vi "syncDAQ_branch.vi"() -> ()   [LabVIEW 2013]
uses:
  <vilib>/Utility/error.llb/DialogType.ctl
  <vilib>/DAQmx/read.llb/DAQmx Read (Analog 1D DBL 1Chan NSamp).vi
  <vilib>/DAQmx/read.llb/DAQmx Read (Analog 1D Wfm NChan NSamp).vi
  <vilib>/DAQmx/miscellaneous.llb/DAQmx Fill In Error Info.vi
  <vilib>/ErrorRing/Error Ring.xnode
panel:
  in  "Ratio":dbl=0.2 caption="复位时间比"
  in  "Vx_Max":dbl=3.0 caption="X向最大电压"
  in  "Vy_Max":dbl=3.0 caption="Y向最大电压"
  in  "N_x":i32=512 caption="采样行数"
  in  "N_y":i32=512 caption="每行采样数"
  in  "停止按钮":bool
  in  "每次采集行数":i32=16
  in  "physical channels read":tag="Dev1/ai0" caption="物理通道（读取）"
  in  "physical channels write":tag="Dev1/ao0:1" caption="物理通道（写入）"
  out "number of samples\nper channel":i32=10240 caption="每通道采样数"
  in  "timing source":tag="OnboardClock" caption="定时源"
  in  "rate":dbl=250000.0 caption="采样速率" format="%#_6f"
  in  "采样模式":enum32{"有限采样", "连续采样"}(tab)
  out "data read 3":waveform(dbl)[](graph) caption="数据输出"
  out "强度图":dbl[][](graph)
  out "data read":waveform(dbl)[](graph) caption="数据输出"
  out "data write":waveform(dbl)[](graph) caption="数据输出"
  # "Basic DAQ\nsettings"
  # "Imaging settings"
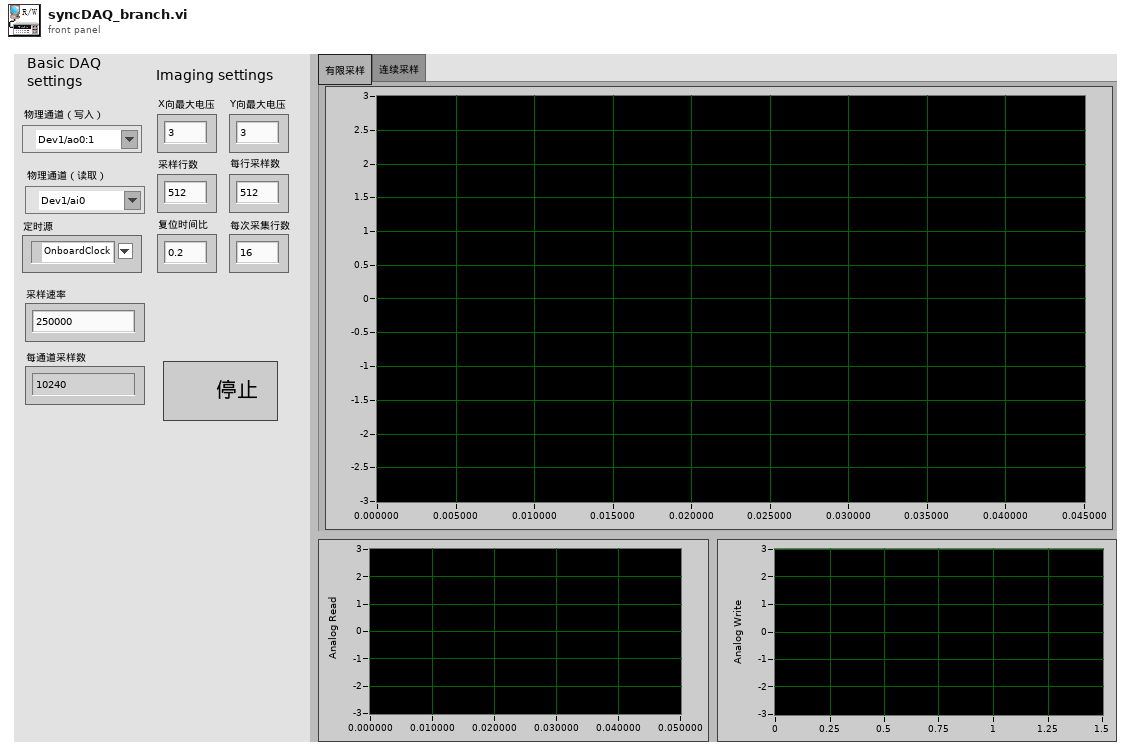
[diagram p1: front panel]
types:
  T1 = cluster{"Vx_Max":dbl, "Vy_Max":dbl, "Tx":dbl, "Row_N":i32, "Ratio":dbl}
  T2 = typedef "DialogType.ctl" = u16
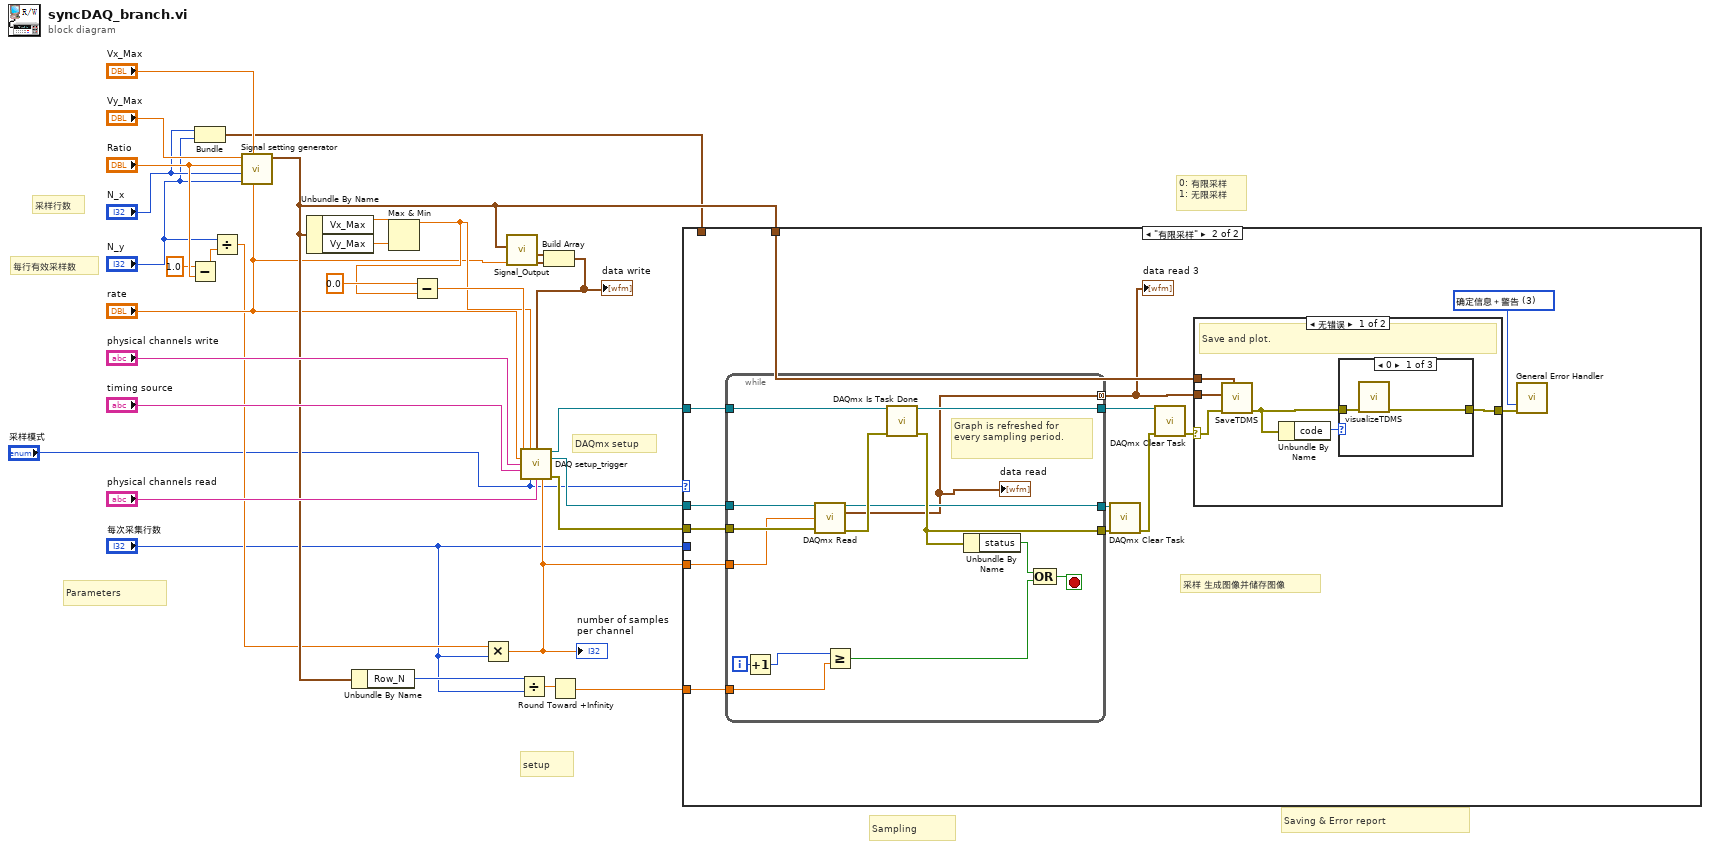
[diagram p0: block diagram]
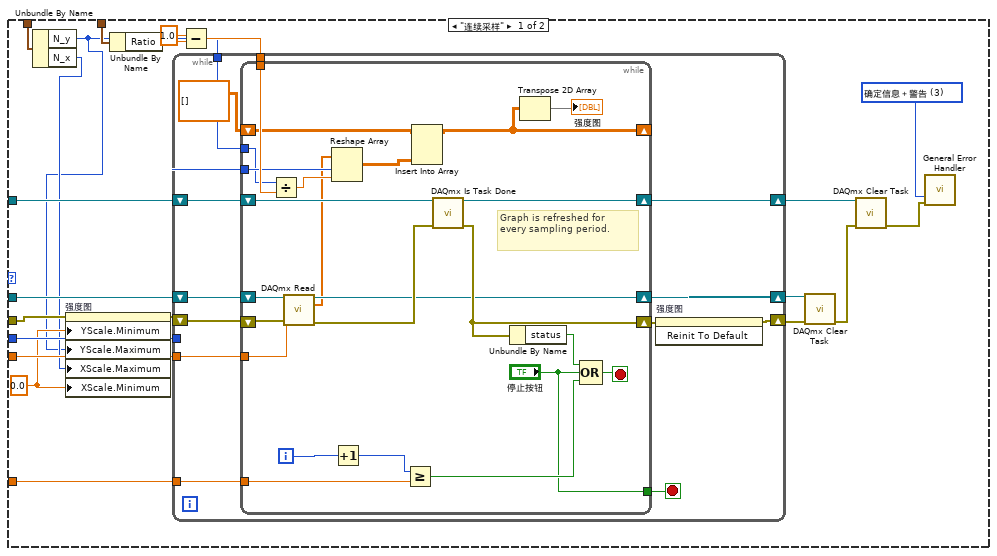
[diagram p2: hidden frame]
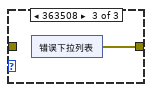
[diagram p4: hidden frame]
diagram:
  # "Saving & Error report"
  # "0: 有限采样\n1: 无限采样"
  # "每行有效采样数"
  # "采样行数"
  # "DAQmx setup"
  # "Parameters"
  # "Sampling"
  # "setup"
  n1 = Subtract(x=1.0, y="Ratio") -> (x-y=w11:dbl)
  n2 = Bundle("N_x"="N_x", "N_y"="N_y") -> (w2:cluster{"N_x":i32, "N_y":i32})  [unwired: 1 in]
  n3 = Divide(x="N_y", y=w11) -> (x/y=w10:dbl)
  n4 = call "Signal setting generator.vi"("rate"="rate", "Vx_Max"="Vx_Max", "N_y"="N_y", "N_x"="N_x", "Ratio"="Ratio", "Vy_Max"="Vy_Max") -> ("Waveform out"=w18:T1)  [unwired: 5 in]
  n5 = Unbundle By Name(w18) -> ("Vx_Max"=w21:dbl, "Vy_Max"=w20:dbl)
  n6 = Unbundle By Name(w18) -> ("Row_N"=w8:i32)
  n7 = Max & Min(x=w21, y=w20) -> (max(x,y)=w19:dbl)  [unwired: 1 out]
  n8 = Subtract(x=0.0, y=w19) -> (x-y=w26:dbl)
  n9 = Multiply(x=w10, y="每次采集行数") -> (x*y=w14:dbl)
  "number of samples\nper channel" <- w14
  n10 = call "Signal_Output.vi"("Fs (Hz)"="rate", "Waveform settings"=w18) -> ("Y"=w22:waveform(dbl), "X"=w23:waveform(dbl))  [unwired: 7 in, 1 out]
  n11 = Divide(x=w8, y="每次采集行数") -> (x/y=w7:dbl)
  n12 = Build Array(w23, w22) -> (w9:waveform(dbl)[])
  "data write" <- w9
  n13 = call "DAQ setup_trigger.vi"("Vx_min"=w26, "Vx_max"=w19, "数组"=w9, "rate"="rate", "physical channels write"="physical channels write", "Timing source"="timing source", "sample mode"="采样模式", "physical channels read"="physical channels read", "Number of samples per channel"=w14) -> ("Writing task out"=w31:refnum<k21>, "Reading task out"=w30:refnum<k21>, "错误输出"=w29:errorcluster)  [unwired: 4 in]
  n14 = Round Toward +Infinity(x=w7) -> (ceil(x): smallest int >= x=w6:dbl)
  n15 = case shown="\"有限采样\"" "采样模式" {
    tunnel: w31 -> [w52 w104]
    tunnel: w30 -> [w46 w98]
    tunnel: w29 -> [w36 w97]
    tunnel: w18 -> [w41 w94]
    tunnel: w14 -> [w45 w93]
    tunnel: w6 -> [w44 w91]
    tunnel: w2 -> [w40 _]
    tunnel: "每次采集行数" -> [w42 _]
    frame "连续采样" {
      w34 = 0.0 ("X标尺.范围:最小值")
      w47 = T2 3 items=["无对话框", "确定信息", "继续或停止信息", "确定信息＋警告", "继续/停止+警告"] ("type of dialog (OK msg:1)")
      n16 = Unbundle By Name(w40) -> ("N_y"=w32:i32, "N_x"=w33:i32)
      n17 = property on="强度图" class="IntGraph (严格)"(error in=w36, "YScale.Minimum"=w34, "YScale.Maximum"=w32, "XScale.Maximum"=w33, "XScale.Minimum"=w34) -> (error out=w35:errorcluster)  [unwired: 1 in, 1 out]
      n18 = Unbundle By Name(w41) -> ("Ratio"=w39:dbl)
      n19 = Subtract(x=1.0, y=w39) -> (x-y=w38:dbl)
      n20 = while {
        tunnel: w45 -> [w62]
        tunnel: w44 -> [w61]
        tunnel: w42 -> [w59]
        tunnel: w38 -> [w58]
        shift-right: [w57] -> w49
        shift-left: w52 -> [w66]
        shift-right: [w65] -> w51
        shift-left: w46 -> [w64]
        shift-right: [w53] -> w50
        shift-left: w35 -> [w63]
        tunnel: w32 -> [w56]
        stop <- w60 stop-if-true
        n21 = while {
          tunnel: w62 -> [w85]
          tunnel: w61 -> [w82]
          shift-right: [w68] -> _
          shift-left: dbl[][] [] -> [w72]
          tunnel: ["停止按钮"] -> w60
          tunnel: w59 -> [w74]
          tunnel: w58 -> [w76]
          shift-right: [w75] -> w57
          shift-left: w66 -> [w78]
          shift-right: [w88] -> w65
          shift-left: w64 -> [w86]
          shift-right: [w89] -> w54
          shift-left: w63 -> [w87]
          tunnel: w56 -> [w70]
          i -> [w77]
          stop <- w80 stop-if-true
          # "Graph is refreshed for\nevery sampling period."
          n22 = Divide(x=w70, y=w76) -> (x/y=w73:dbl)
          n23 = call-poly <vilib>:"DAQmx Read.vi"("task/channels in"=w86, "number of samples per channel"=w85, "error in"=w87) -> ("task out"=w88:refnum<k21>, "data"=w67:dbl[], "error out"=w90:errorcluster)  [unwired: 10 in]
          n24 = Reshape Array(w67, w74, w73) -> (w71:dbl[][])
          n25 = Increment(x=w77) -> (x+1=w83:i32)
          n26 = Greater Or Equal?(x=w83, y=w82) -> (x >= y?=w81:bool)
          n27 = Insert Into Array(array=w72, new element=w71) -> (w68:dbl[][])  [unwired: 2 in]
          n28 = call <vilib>:"DAQmx Is Task Done.vi"("task/channels in"=w78, "error in"=w90) -> ("task out"=w75:refnum<k21>, "error out"=w89:errorcluster)  [unwired: 11 in, 1 out]
          n29 = Unbundle By Name(w89) -> ("status"=w84:bool)
          n30 = Transpose 2D Array(2D array=w68) -> (transposed array=→"强度图":dbl[][])
          n31 = Compound Arithmetic op=OR(w84, "停止按钮", w81) -> (w80:bool)
        }
        n32 = invoke on="强度图" class="IntGraph (严格)" method="Reinit To Default"(error in=w54) -> (error out=w53:errorcluster)  [unwired: 2 in, 2 out]
      }
      n33 = call <vilib>:"DAQmx Clear Task.vi"("task in"=w51, "error in"=w50) -> ("error out"=w48:errorcluster)  [unwired: 13 in]
      n34 = call <vilib>:"DAQmx Clear Task.vi"("task in"=w49, "error in"=w48) -> ("error out"=w43:errorcluster)  [unwired: 13 in]
      n35 = call <vilib>:"General Error Handler.vi"("type of dialog (OK msg:1)"=w47, "error in (no error)"=w43) -> ()  [unwired: 9 in, 5 out]
    }
    frame "有限采样" {
      w99 = T2 3 items=["无对话框", "确定信息", "继续或停止信息", "确定信息＋警告", "继续/停止+警告"] ("type of dialog (OK msg:1)")
      # "采样 生成图像并储存图像"
      n36 = while {
        tunnel: w98 -> [w125]
        tunnel: w104 -> [w128]
        tunnel: w97 -> [w126]
        tunnel: [w130] -> w102
        tunnel: [w129] -> w103
        tunnel: [w127] -> w101
        tunnel: w93 -> [w124]
        tunnel: w91 -> [w119]
        tunnel: [w117] -> w92 mode=concatenating
        i -> [w121]
        stop <- w123 stop-if-true
        # "Graph is refreshed for\nevery sampling period."
        n37 = Increment(x=w121) -> (x+1=w120:i32)
        n38 = call-poly <vilib>:"DAQmx Read.vi"("task/channels in"=w125, "number of samples per channel"=w124, "error in"=w126) -> ("task out"=w129:refnum<k21>, "data"=w117:waveform(dbl)[], "error out"=w131:errorcluster)  [unwired: 10 in]
        "data read" <- w117
        n39 = Greater Or Equal?(x=w120, y=w119) -> (x >= y?=w118:bool)
        n40 = call <vilib>:"DAQmx Is Task Done.vi"("task/channels in"=w128, "error in"=w131) -> ("task out"=w127:refnum<k21>, "error out"=w130:errorcluster)  [unwired: 11 in, 1 out]
        n41 = Unbundle By Name(w130) -> ("status"=w122:bool)
        n42 = Compound Arithmetic op=OR(w122, w118) -> (w123:bool)
      }
      "data read 3" <- w92
      n43 = call <vilib>:"DAQmx Clear Task.vi"("task in"=w103, "error in"=w102) -> ("error out"=w100:errorcluster)  [unwired: 13 in]
      n44 = call <vilib>:"DAQmx Clear Task.vi"("task in"=w101, "error in"=w100) -> ("error out"=w95:errorcluster)  [unwired: 13 in]
      n45 = case "条件结构" shown="无错误" w95 {
        selector: w95 -> [w109 w116]
        tunnel: w92 -> [w110 _]
        tunnel: [w106 w116] -> w96
        tunnel: w94 -> [w105 _]
        frame No Error {
          # "Save and plot."
          n46 = call "SaveTDMS.vi"("Waveform settings"=w105, "错误输入（无错误）"=w109, "数据"=w110) -> ("错误输出"=w108:errorcluster)  [unwired: 8 in]
          n47 = Unbundle By Name(w108) -> ("code"=w107:i32)
          n48 = case shown="0" w107 {
            tunnel: w108 -> [w112 w113 _]
            tunnel: [w111 w113 w114] -> w106
            frame 0 {
              n49 = call "visualizeTDMS.vi"("错误输入（无错误）"=w112) -> ("错误输出"=w111:errorcluster)  [unwired: 8 in, 2 out]
            }
            frame Default {
            }
            frame 363508 {
              n50 = xnode "错误下拉列表"() -> ("错误输出"=w114:errorcluster)
            }
          }
        }
        frame Error {
        }
      }
      n51 = call <vilib>:"General Error Handler.vi"("type of dialog (OK msg:1)"=w99, "error in (no error)"=w96) -> ()  [unwired: 9 in, 5 out]
    }
  }
